vi "AddPoint.vi"(4 "FlipY":bool, 6 "FlipX":bool, 8 "error in (no error)":errorcluster, 9 "Pixels":i32[](array[numeric]), 10 "?":T1={"Calibration Input"=[], "CalibrationResults"={"Center in Pixels"=[374.0120339529387, 375.46592887074246], "Angle"=0.022945275255000355, "Pixels/MHz X"=0.0, "Pixels/MHz Y"=0.0}, "Highlight"=[], "Running Script"=refnum}, 11 "Cluster":T2) -> (0 "error out":errorcluster)   [LabVIEW 2017]
uses:
  TypeDefinitions/SubVIQueues.ctl
  AODControl/MessageQueue/QueueOperations/All Message Queues.ctl
  AODControl/MessageQueue/QueueOperations/Message Cluster.ctl
  TypeDefinitions/ExperimentVariables.ctl
  AODControl/AODControlFiles/AODPointDefinition.ctl
  MessageQueue/QueueOperations/Enqueue Message (Single).vi
  MessageQueue/MessageQueue.lvlib
  AODControl/AODControl.lvlib
  AODControl/MessageQueue/MessageQueue.lvlib
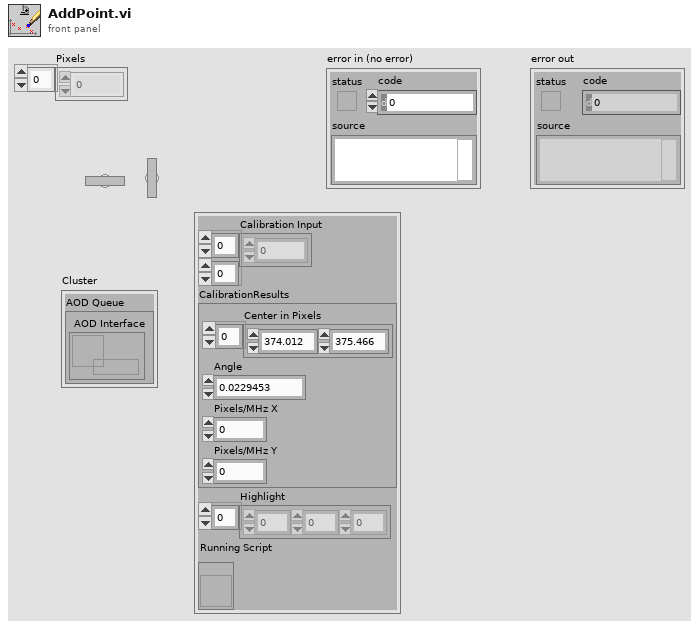
[diagram p1: front panel]
types:
  T1 = typedef "ExperimentVariables.ctl" = cluster{"Calibration Input":i32[][], "CalibrationResults":cluster{"Center in Pixels":dbl[], "Angle":dbl, "Pixels/MHz X":dbl, "Pixels/MHz Y":dbl}, "Highlight":i32[], "Running Script":refnum<vi>}
  T2 = typedef "SubVIQueues.ctl" = cluster{"AOD Queue":T3}
  T3 = typedef "AODControl.lvlib/MessageQueue.lvlib/All Message Queues.ctl" = cluster{" AOD Interface":refnum<queue>}
  T4 = typedef "AODControl.lvlib/AODPointDefinition.ctl" = cluster{"Freq X":dbl, "Freq Y":dbl, "Index":i32, "Ampitude":dbl}
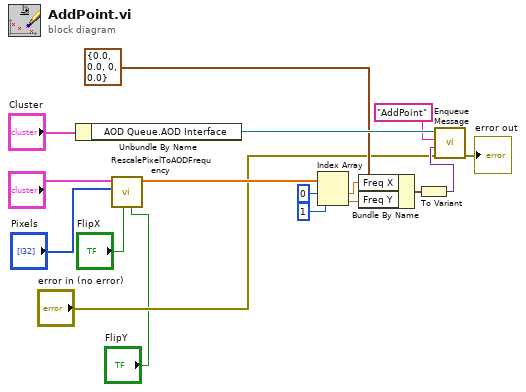
[diagram p0: block diagram]
diagram:
  n1 = Unbundle By Name("Cluster") -> ("AOD Queue.AOD Interface"=w17:refnum<queue>)
  n2 = call "RescalePixelToAODFrequency.vi"("FlipY"="FlipY", "FlipX"="FlipX", "Pixels"="Pixels", 11:"?") -> ("Array"=w9:dbl[])  [unwired: 7 in]
  n3 = Index Array(array=w9, index #1=0 ("index"), index #2=1 ("index")) -> (element #1=w13:dbl, element #2=w12:dbl)
  n4 = Bundle By Name(cluster=T4 {"Freq X"=0.0, "Freq Y"=0.0, "Index"=0, "Ampitude"=0.0} ("Cluster"), "Freq X"=w13, "Freq Y"=w12) -> (w11:T4)
  n5 = To Variant(anything=w11) -> (Variant=w10:variant)
  n6 = call-poly "Enqueue Message.vi"("error in (no error)"="error in (no error)", "Message Data"=w10, "Message"="AddPoint", "Message Queue"=w17) -> ("error out"=→"error out":errorcluster)  [unwired: 6 in, 1 out]
